vi "Edit Step.vi"(0 "Script in":T3, 5 "new element/subarray":T1={"Direction"=enum."Chamber", "Pressure MPa"=0.0, "Time s"=0.0, "Delta alarm MPa"=0.0, "Delta warning MPa"=0.0}, 7 "index":i32) -> (4 "Script out":T3)   [LabVIEW 2019]
uses:
  TypeDef/Script.ctl
  TypeDef/Step.ctl
  TypeDef/Direction.ctl
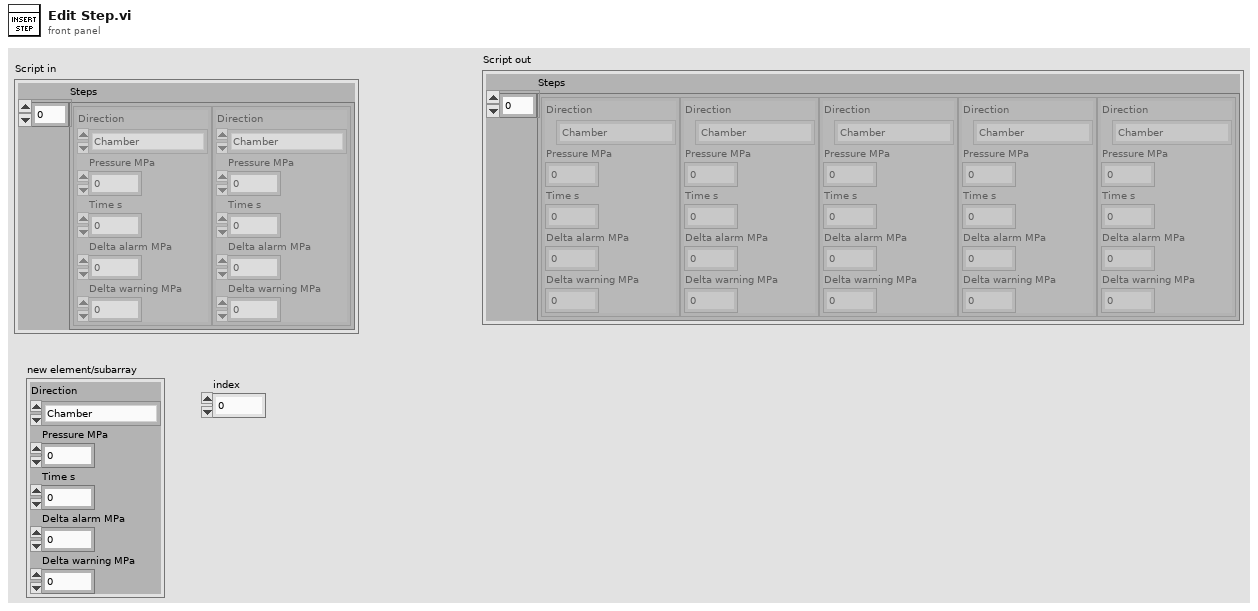
[diagram p1: front panel]
types:
  T1 = typedef "Step.ctl" = cluster{"Direction":T2, "Pressure MPa":dbl, "Time s":dbl, "Delta alarm MPa":dbl, "Delta warning MPa":dbl}
  T2 = typedef "Direction.ctl" = enum16{"None", "DUT", "Chamber"}
  T3 = typedef "Script.ctl" = cluster{"Steps":T1[]}
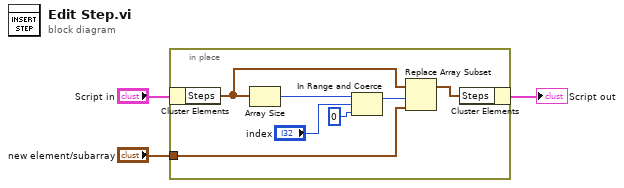
[diagram p0: block diagram]
diagram:
  n1 = in-place {
    in-place-border: "new element/subarray" -> [w9]
    n2 = in-place-cluster #1("Script in") -> ("Steps"=w6:T1[])
    n3 = Array Size(array=w6) -> (size(s)=w5:i32)
    n4 = In Range and Coerce(upper limit=w5, x="index", lower limit=0) -> (coerced(x)=w4:i32)  [unwired: 1 out]
    n5 = Replace Array Subset(array=w6, new element=w9, index=w4) -> (w10:T1[])
    n6 = in-place-cluster #1("Steps"=w10) -> (→"Script out":T3)
  }
